vi "Drive_data.vi"(10 "Drive sensor data":T2={"Left drive encoder"=0.0, "Right drive encoder"=0.0, "Left shift switch"=TRUE, "Right shift switch"=TRUE, "Gyro"=0.0}, 11 "Drive output commands":T3={"Left drive power"=0.0, "Right drive power"=0.0, "Left shift"=TRUE, "Right shift"=TRUE}) -> (3 "Subsystem data out":T1={"Subsystem name"="Drive", "Double data points"=[], "Boolean data points"=[], "Boolean channel names"=[], "Double channel names"=[]})   [LabVIEW 2017, in "labview-standard-library.lvlib"]
uses:
  labview-standard-library.lvlib
  universial-controls/Drive_commands_global.ctl
  universial-controls/Drive_sensors_global.ctl
  Subsystem_data.ctl
  universial-controls/Drive_TDMS_channel_names.ctl
panel:
  in  "Subsystem data in":T1={"Subsystem name"="Drive", "Double data points"=[], "Boolean data points"=[], "Boolean channel names"=[], "Double channel names"=[]}
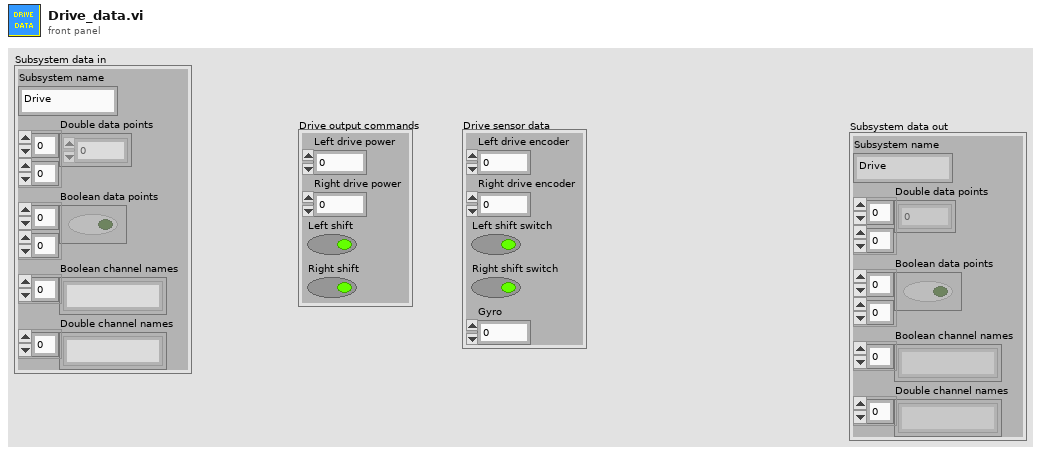
[diagram p1: front panel]
types:
  T1 = typedef "labview-standard-library.lvlib/Subsystem_data.ctl" = cluster{"Subsystem name":string, "Double data points":dbl[][], "Boolean data points":bool[][], "Boolean channel names":string[], "Double channel names":string[]}
  T2 = typedef "labview-standard-library.lvlib/Drive_sensors_global.ctl" = cluster{"Left drive encoder":dbl, "Right drive encoder":dbl, "Left shift switch":bool, "Right shift switch":bool, "Gyro":dbl}
  T3 = typedef "labview-standard-library.lvlib/Drive_commands_global.ctl" = cluster{"Left drive power":dbl, "Right drive power":dbl, "Left shift":bool, "Right shift":bool}
  T4 = typedef "labview-standard-library.lvlib/Drive_TDMS_channel_names.ctl" = cluster{"Boolean":string[], "Double":string[]}
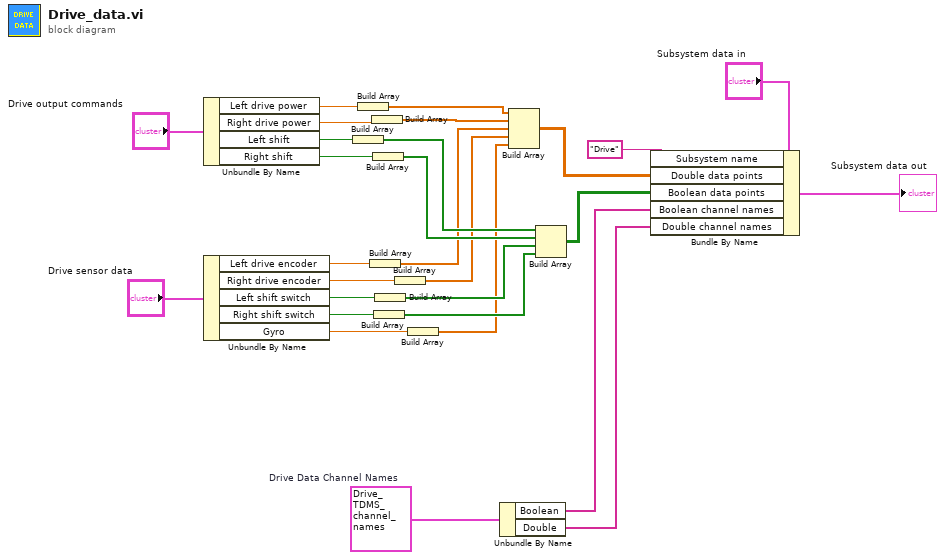
[diagram p0: block diagram]
diagram:
  w17 = T4 {"Boolean"=["Left_shift", "Right_shift", "Left_shift_switch", "Right_shift_switch", ""], "Double"=["Left_drive_power", "Right_drive_power", "Left_drive_encoder", "Right_drive_encoder", "Gyro"]}  # Drive Data Channel Names
  n1 = Unbundle By Name("Drive output commands") -> ("Left drive power"=w26:dbl, "Right drive power"=w25:dbl, "Left shift"=w21:bool, "Right shift"=w20:bool)
  n2 = Unbundle By Name("Drive sensor data") -> ("Left drive encoder"=w24:dbl, "Right drive encoder"=w23:dbl, "Left shift switch"=w19:bool, "Right shift switch"=w18:bool, "Gyro"=w22:dbl)
  n3 = Build Array(w21) -> (w7:bool[])
  n4 = Build Array(w26) -> (w9:dbl[])
  n5 = Build Array(w24) -> (w5:dbl[])
  n6 = Build Array(w25) -> (w8:dbl[])
  n7 = Build Array(w20) -> (w6:bool[])
  n8 = Build Array(w18) -> (w2:bool[])
  n9 = Build Array(w19) -> (w3:bool[])
  n10 = Build Array(w23) -> (w4:dbl[])
  n11 = Build Array(w22) -> (w1:dbl[])
  n12 = Unbundle By Name(w17) -> ("Boolean"=w11:string[], "Double"=w10:string[])
  n13 = Build Array(w9, w8, w5, w4, w1) -> (w13:dbl[][])
  n14 = Build Array(w7, w6, w3, w2) -> (w12:bool[][])
  n15 = Bundle By Name(cluster="Subsystem data in", "Subsystem name"="Drive", "Double data points"=w13, "Boolean data points"=w12, "Boolean channel names"=w11, "Double channel names"=w10) -> (→"Subsystem data out":T1)
